vi "Append Popup.vi"(7 "Column":i32, 8 "error in (no error)":errorcluster caption="错误输入（无错误）", 9 "RangText":string[](array[string]), 10 "PopupRef":refnum<vi>, 11 "Popup 输入":refnum<class "Popup.lvclass"> caption="DNL_LabVIEW Object in") -> (0 "error out":errorcluster caption="错误输出", 3 "Popup 输出":refnum<class "Popup.lvclass"> caption="DNL_LabVIEW Object out")   [LabVIEW 2017, in "Popup.lvclass"]
uses:
  Popup.lvclass
  Popup.lvclass/Popup.ctl
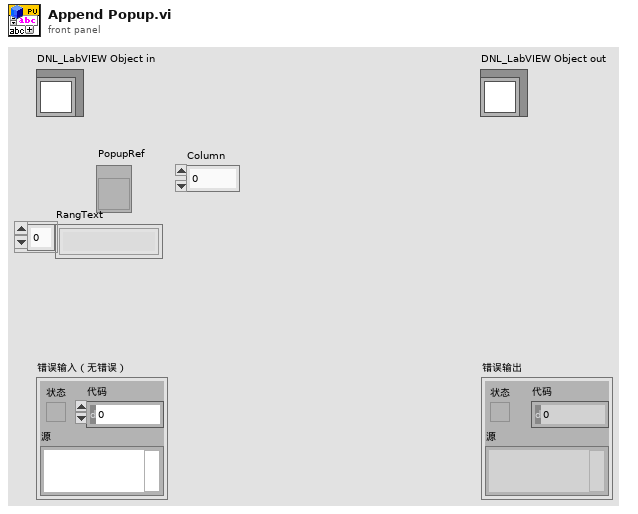
[diagram p1: front panel]
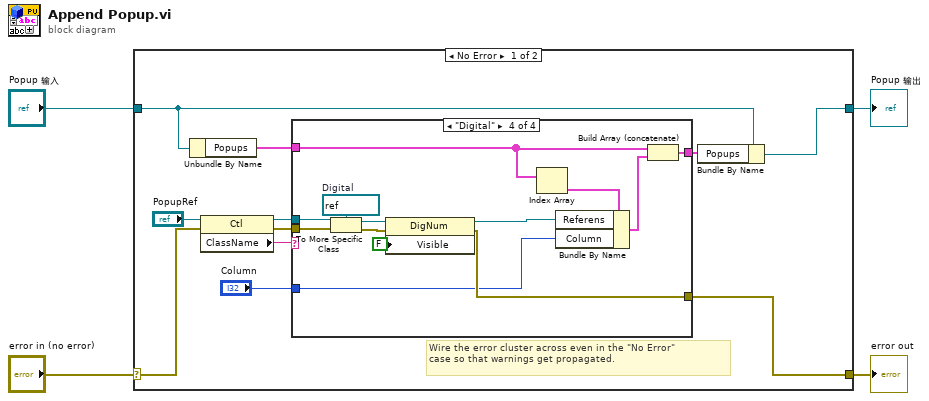
[diagram p0: block diagram]
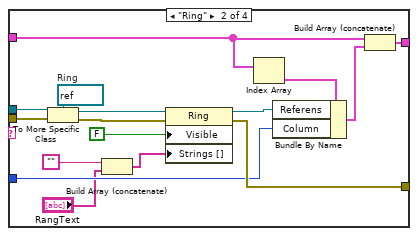
[diagram p3: hidden frame]
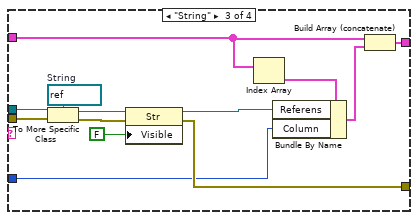
[diagram p4: hidden frame]
diagram:
  n1 = case shown="No Error" "error in (no error)" {
    selector: "error in (no error)" -> [w10 w61]
    tunnel: [w6 w61] -> w3
    tunnel: [w15 w60] -> w1
    tunnel: "Popup 输入" -> [w14 w60]
    frame No Error {
      # "Wire the error cluster across even in the \"No Error\"\ncase so that warnings get propagated."
      n2 = Unbundle By Name(w14) -> ("Popups"=w13:cluster{"Referens":refnum<vi>, "Column":i32}[])
      n3 = property class="Ctl"(reference="PopupRef", error in=w10) -> (reference out=w8:refnum<vi>, error out=w7:errorcluster, "ClassName"=w9:string)
      n4 = case shown="\"Digital\"" w9 {
        tunnel: w13 -> [w17 w32 w45 w58]
        tunnel: [w17 w30 w43 w56] -> w12
        tunnel: w8 -> [_ w28 w41 w54]
        tunnel: w7 -> [w16 w29 w42 w55]
        tunnel: [w16 w22 w35 w48] -> w6
        tunnel: "Column" -> [_ w21 w34 w47]
        frame "假", Default {
        }
        frame "Ring" {
          w27 = refnum<vi> refnum  # Ring
          n5 = To More Specific Class(target class=w27, reference=w28, error in=w29) -> (specific class reference=w26:refnum<vi>, error out=w25:errorcluster)
          n6 = Build Array (concatenate)("", "RangText") -> (w18:string[])
          n7 = property class="Ring"(reference=w26, error in=w25, "Visible"=FALSE, "Strings []"=w18) -> (reference out=w24:refnum<vi>, error out=w22:errorcluster)
          n8 = Index Array(array=w32) -> (element=w33:cluster{"Referens":refnum<vi>, "Column":i32})  [unwired: 1 in]
          n9 = Bundle By Name(cluster=w33, "Referens"=w24, "Column"=w21) -> (w31:cluster{"Referens":refnum<vi>, "Column":i32})
          n10 = Build Array (concatenate)(w32, w31) -> (w30:cluster{"Referens":refnum<vi>, "Column":i32}[])
        }
        frame "String" {
          w40 = refnum<vi> refnum  # String
          n11 = To More Specific Class(target class=w40, reference=w41, error in=w42) -> (specific class reference=w39:refnum<vi>, error out=w38:errorcluster)
          n12 = property class="Str"(reference=w39, error in=w38, "Visible"=FALSE) -> (reference out=w37:refnum<vi>, error out=w35:errorcluster)
          n13 = Index Array(array=w45) -> (element=w46:cluster{"Referens":refnum<vi>, "Column":i32})  [unwired: 1 in]
          n14 = Bundle By Name(cluster=w46, "Referens"=w37, "Column"=w34) -> (w44:cluster{"Referens":refnum<vi>, "Column":i32})
          n15 = Build Array (concatenate)(w45, w44) -> (w43:cluster{"Referens":refnum<vi>, "Column":i32}[])
        }
        frame "Digital" {
          w53 = refnum<vi> refnum  # Digital
          n16 = To More Specific Class(target class=w53, reference=w54, error in=w55) -> (specific class reference=w52:refnum<vi>, error out=w51:errorcluster)
          n17 = property class="DigNum"(reference=w52, error in=w51, "Visible"=FALSE) -> (reference out=w50:refnum<vi>, error out=w48:errorcluster)
          n18 = Index Array(array=w58) -> (element=w59:cluster{"Referens":refnum<vi>, "Column":i32})  [unwired: 1 in]
          n19 = Bundle By Name(cluster=w59, "Referens"=w50, "Column"=w47) -> (w57:cluster{"Referens":refnum<vi>, "Column":i32})
          n20 = Build Array (concatenate)(w58, w57) -> (w56:cluster{"Referens":refnum<vi>, "Column":i32}[])
        }
      }
      n21 = Bundle By Name(cluster=w14, "Popups"=w12) -> (w15:refnum<class "Popup.lvclass">)
    }
    frame Error {
    }
  }
  "error out" <- w3
  "Popup 输出" <- w1
